vi "Part Name IA.vi"(8 "error in (no error)":errorcluster, 10 "Part Name":string, 11 "Image Acquisition in":refnum<class "Image Acquisition.lvclass">) -> (0 "error out":errorcluster, 3 "Image Acquisition out":refnum<class "Image Acquisition.lvclass">)   [LabVIEW 2019, in "Image Acquisition.lvlib" / "Image Acquisition.lvclass"]
uses:
  Image Acquisition.lvclass
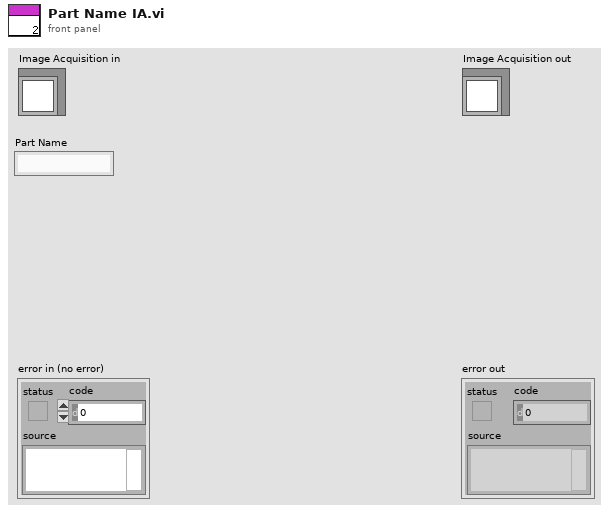
[diagram p1: front panel]
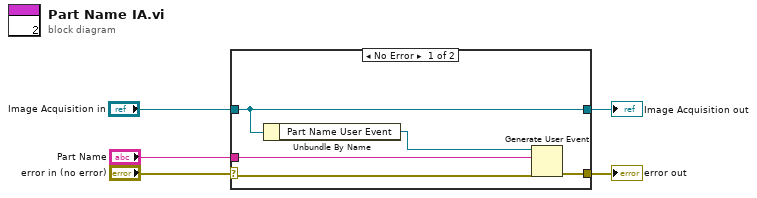
[diagram p0: block diagram]
diagram:
  n1 = case shown="No Error" "error in (no error)" {
    selector: "error in (no error)" -> [w10 w12]
    tunnel: [w9 w12] -> w4
    tunnel: [w8 w11] -> w2
    tunnel: "Image Acquisition in" -> [w8 w11]
    tunnel: "Part Name" -> [w6 _]
    frame No Error {
      n2 = Unbundle By Name(w8) -> ("Part Name User Event"=w7:refnum<user-event>)
      n3 = Generate User Event(user event=w7, event data cluster=w6, error in=w10) -> (error out=w9:errorcluster)  [unwired: 1 in, 1 out]
    }
    frame Error {
    }
  }
  "error out" <- w4
  "Image Acquisition out" <- w2
